vi "new encoder sampling trial.vi"() -> ()   [LabVIEW 2018]
uses:
  <vilib>/ptbypt/NI_PtbyPt.lvlib
panel:
  in  "amplitude":dbl=1.0 format="%#_13g"
  out "Waveform Graph":dbl[][](graph)
  in  "speed (Hz)":dbl=666.0 format="%#_13g"
  in  "filter torque":bool
  in  "switch encoders":bool
  in  "rising edge (T)":bool
  out "ticks out":u32[](array[numeric])
  in  "STOP":bool=TRUE
  out "Waveform Chart":T1(graph)
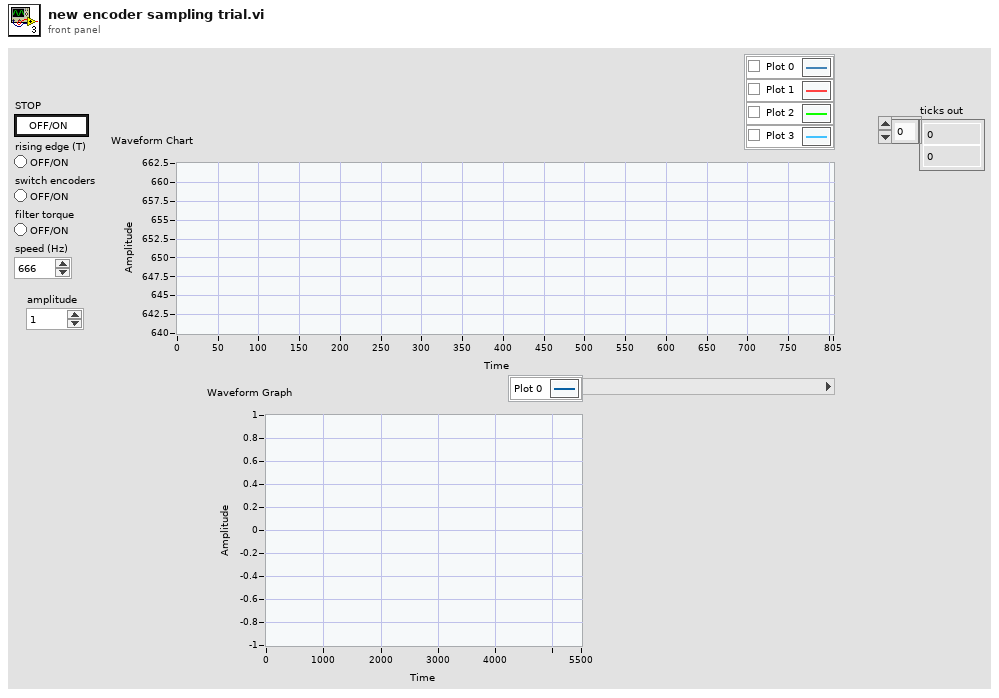
[diagram p1: front panel]
types:
  T1 = cluster{sgl, "calculated speed (rad/tick)":sgl, sgl, "calculated angle (radians)":sgl}
  T2 = cluster{sgl, "calculated speed (rad/tick)":sgl, sgl, "calculated angle (radians)":sgl}[]
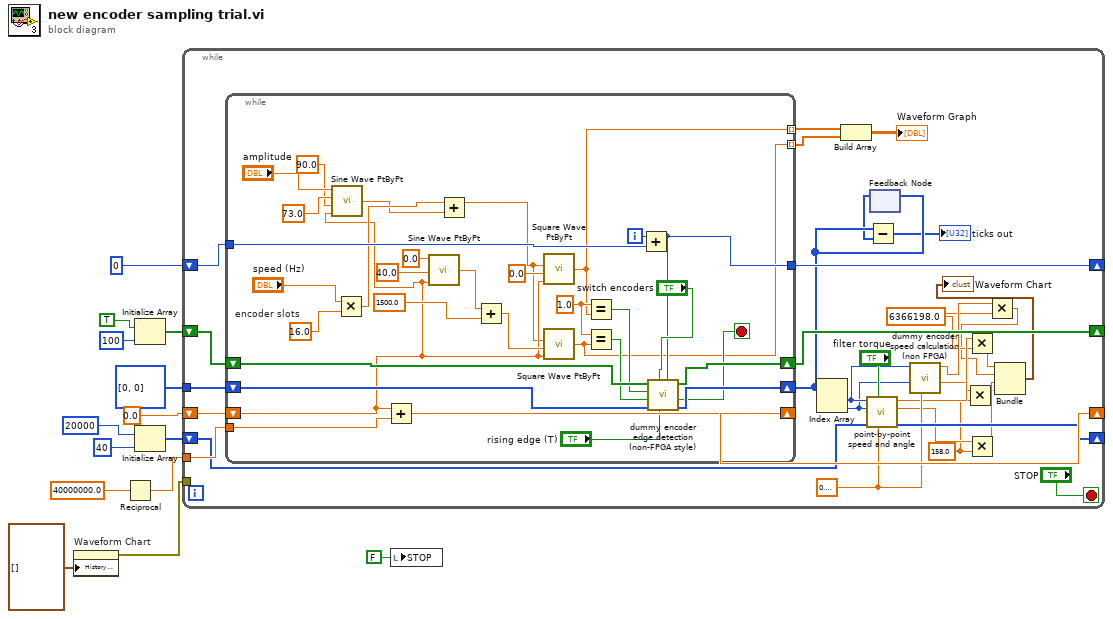
[diagram p0: block diagram]
diagram:
  n1 = property on="Waveform Chart" class="WFChart (strict)"("History Data"=T2 []) -> (error out=w4:errorcluster)  [unwired: 2 in, 1 out]
  n2 = Reciprocal(x=40000000.0 ("frequency")) -> (1/x=w9:dbl)
  n3 = Initialize Array(TRUE, 100 ("dimension size")) -> (w11:bool[])
  n4 = Initialize Array(u32 20000, 40 ("dimension size")) -> (w7:u32[])
  n5 = while {
    tunnel: u32[] [0, 0] ("ticks") -> [w46]
    tunnel: w9 -> [w43]
    shift-right: [w41] -> _
    shift-left: 0.0 ("frequency") -> [w42]
    shift-right: [w38] -> _
    shift-left: w7 -> [w39]
    shift-right: [w37] -> _
    shift-left: w11 -> [w45]
    tunnel: w4 -> [_]
    shift-right: [w36] -> _
    shift-left: u32 0 ("dimension size") -> [w35]
    stop <- "STOP" stop-if-true
    w15 = sgl 158.0 ("y")
    w19 = sgl 6366198.0 ("x")
    w32 = sgl 0.3 ("encoder fixed offest")
    n6 = while {
      shift-right: [w76] -> w41
      shift-left: w42 -> [w53]
      shift-right: [w65] -> w25
      shift-left: w46 -> [w66]
      shift-right: [w64] -> w37
      shift-left: w45 -> [w69]
      tunnel: w43 -> [w77]
      tunnel: [w59] -> w36
      tunnel: w35 -> [w58]
      tunnel: [w48] -> w28 mode=indexing
      tunnel: [w47] -> w27 mode=indexing
      i -> [w60]
      stop <- w63 stop-if-true
      w57 = 16.0  # encoder slots
      w75 = 1.0 ("x")
      n7 = call <vilib>:"Sine Wave PtByPt.vi"("time"=w53, "phase"=90.0, "frequency"=73.0, "amplitude"="amplitude") -> ("sine wave"=w51:dbl)
      n8 = Multiply(x="speed (Hz)", y=w57) -> (x*y=w56:dbl)
      n9 = Add(x=w53, y=w77) -> (x+y=w76:dbl)
      n10 = call <vilib>:"Sine Wave PtByPt.vi"("time"=w53, "frequency"=40.0, "amplitude"=0.0) -> ("sine wave"=w72:dbl)  [unwired: 1 in]
      n11 = Add(x=w56, y=w51) -> (x+y=w52:dbl)
      n12 = Add(x=w72, y=1500.0 ("phase")) -> (x+y=w70:dbl)
      n13 = call <vilib>:"Square Wave PtByPt.vi"("frequency"=w52, "phase"=0.0, "time"=w53) -> ("square wave"=w48:dbl)  [unwired: 2 in]
      n14 = call <vilib>:"Square Wave PtByPt.vi"("frequency"=w52, "phase"=w70, "time"=w53) -> ("square wave"=w47:dbl)  [unwired: 2 in]
      n15 = Equal?(x=w75, y=w48) -> (x = y?=w68:bool)
      n16 = Equal?(x=w75, y=w47) -> (x = y?=w67:bool)
      n17 = Add(x=w60, y=w58) -> (x+y=w59:u32)
      n18 = call "dummy encoder edge detection (non-FPGA style).vi"("Tick Count(Ticks)"=w59, "rising edge (T)"="rising edge (T)", "switch encoders (F)"="switch encoders", "ticks"=w66, "encoder 2"=w67, "encoder 1"=w68, "history in"=w69) -> ("ticks out"=w65:u32[], "edge detected"=w63:bool, "history out"=w64:bool[])  [unwired: 2 in]
    }
    n19 = Index Array(array=w25) -> (element #1=w34:u32, element #2=w33:u32)  [unwired: 2 in]
    n20 = Build Array(w28, w27) -> (→"Waveform Graph":dbl[][])
    n21 = call "point-by-point speed and angle.vi"("encoder fixed offest"=w32, "filter torque"="filter torque", "speed history in"=w39, "angle pulse"=w33, "speed pulse"=w34) -> ("speed history out"=w38:u32[], "calculated angle (radians)"=w30:sgl, "calculated speed (rad/tick)"=w31:sgl)  [unwired: 4 in]
    n22 = feedback-in #1(w25) -> ()
    n23 = feedback #1() -> (w24:u32[])  [unwired: 1 in]
    n24 = Subtract(x=w25, y=w24) -> (x-y=→"ticks out":u32[])
    n25 = call "dummy encoder speed calculation (non FPGA).vi"("encoder fixed offest"=w32, "angle pulse"=w33, "speed pulse"=w34) -> ("calculated angle (radians)"=w22:sgl, "calculated speed (rad/tick)"=w20:sgl)  [unwired: 7 in]
    n26 = Multiply(x=w22, y=w15) -> (x*y=w16:sgl)
    n27 = Multiply(x=w31, y=w19) -> (x*y=w21:sgl)
    n28 = Multiply(x=w30, y=w15) -> (x*y=w17:sgl)
    n29 = Multiply(x=w20, y=w19) -> (x*y=w18:sgl)
    n30 = Bundle(w21, w18, w17, w16) -> (→"Waveform Chart":cluster{sgl, sgl, sgl, sgl})  [unwired: 1 in]
  }
  n31 = local write "STOP"(FALSE ("STOP")) -> ()
